vi "TCP IP Command Tester.vi"() -> ()   [LabVIEW 2024]
uses:
  Controls/Control_Fornax Set Monopolar Command - Coag Mode Enum.ctl
  Controls/Control_Fornax Set Monopolar Command - Serial Number String.ctl
  Controls/Control_Fornax Set Monopolar Command - Energy Channel ID Enum.ctl
  Controls/Control_Fornax Set Monopolar Command - Cut Mode Enum.ctl
  Controls/Control_Fornax Set Monopolar Command - Cut Power Command Enum.ctl
  Controls/Control_Fornax Set Monopolar Command - Coag Power Command Enum.ctl
  Program Files/National Instruments/LabVIEW 2024/examples/Design Patterns/Queued Message Handler/support/QMH Fundamentals - Message Cluster.ctl
panel:
  in  "Tab Control":enum32{"Page 1", "Page 2"}(tab)
  in  "error in (no error)":errorcluster
  out "output cluster":T1
  out "Array":T2(array[cluster])
  in  "Fornax Executable Path":path=path "C:/Program Files (x86)/Medtronic/Fornax/x86/Fornax.exe"
  in  "Action 1":bool
  in  "ExternalCommCommand":T3(ring)=enum."EXTERNAL_COMM_COMMAND_PAIR_INTEGRATION_TESTOR"
  in  "Stop":bool
  out "Display Message":string="Wait while TCP Connection established"
  in  "Set Monopolar Command":bool
  in  "CoagMode":T4
  in  "Serial Number":T5="T5G00443DX"
  in  "EnergyChannelID":T6
  in  "CutMode":T7
  in  "CutPowerCommand":T8
  in  "CoagPowerCommand":T9
  out "String":string
  in  "Numeric (0-8)":i32
  in  "Send String Command":bool
  out "status":bool
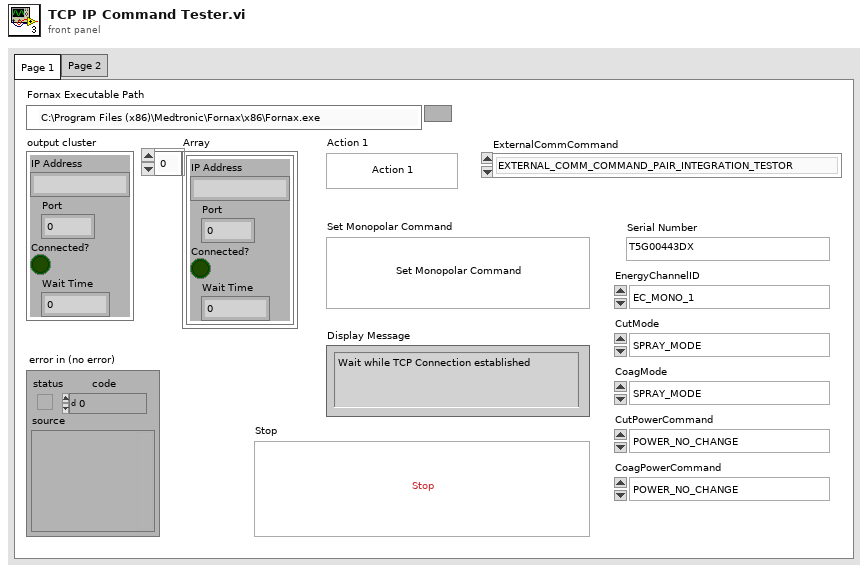
[diagram p1: front panel]
types:
  T1 = cluster{"IP Address":string, "Port":u16, "Connected?":bool, "Wait Time":dbl}
  T2 = cluster{"IP Address":string, "Port":u16, "Connected?":bool, "Wait Time":dbl}[]
  T3 = enum16{"EXTERNAL_COMM_COMMAND_INVALID", "EXTERNAL_COMM_COMMAND_PAIR_VLEX", "EXTERNAL_COMM_COMMAND_PAIR_FORNAX", "EXTERNAL_COMM_COMMAND_PAIR_INTEGRATION_TESTOR", "EXTERNAL_COMM_COMMAND_ENABLE_DFA", "EXTERNAL_COMM_COMMAND_ENABLE_DFT", "EXTERNAL_COMM_COMMAND_ENABLE_VIPER", "EXTERNAL_COMM_COMMAND_AUTO_ETHERNET_ON", "EXTERNAL_COMM_COMMAND_AUTO_ETHERNET_OFF", "EXTERNAL_COMM_COMMAND_STREAM_RFDATA_ON", "EXTERNAL_COMM_COMMAND_STREAM_RFDATA_OFF", "EXTERNAL_COMM_COMMAND_STREAM_ISOFIRM_ON", "EXTERNAL_COMM_COMMAND_STREAM_ISOFIRM_OFF", "EXTERNAL_COMM_COMMAND_STREAM_RFID_ON", "EXTERNAL_COMM_COMMAND_STREAM_RFID_OFF", "EXTERNAL_COMM_COMMAND_AUTO_ETHERNET_ONCE"}
  T4 = typedef "Control_Fornax Set Monopolar Command - Coag Mode Enum.ctl" = enum16{"SPRAY_MODE", "CUT_MODE", "BLEND_MODE", "FULGERATE_MODE", "BEPOLAR_MODE", "VESSEL_SEALING_MODE", "VALLEYLAB_MODE", "BIPOLAR_RESECTION_CUT_MODE", "BIPOLAR_RESECTION_COAG_MODE", "AUTOBIPOLAR_MODE", "VIPER_HLA", "SOFT_COAG_MODE", "NUM_ENERGY_MODES"}
  T5 = typedef "Control_Fornax Set Monopolar Command - Serial Number String.ctl" = string
  T6 = typedef "Control_Fornax Set Monopolar Command - Energy Channel ID Enum.ctl" = enum16{"EC_MONO_1", "EC_BIPOLAR", "EC_MONO_2", "EC_ADVANCED", "NUM_ENERGY_CHANNELS", "EC_NOT_USED"}
  T7 = typedef "Control_Fornax Set Monopolar Command - Cut Mode Enum.ctl" = enum16{"SPRAY_MODE", "CUT_MODE", "BLEND_MODE", "FULGERATE_MODE", "BIPOLAR_MODE", "VESSEL_SEALING_MODE", "VALLEYLAB_MODE", "BIPOLAR_RESECTION_CUT_MODE", "BIPOLAR_RESECTION_COAG_MODE", "AUTOBIPOLAR_MODE", "VIPER_HLA", "SOFT_COAG_MODE", "NUM_ENERGY_MODES"}
  T8 = typedef "Control_Fornax Set Monopolar Command - Cut Power Command Enum.ctl" = enum16{"POWER_NO_CHANGE", "POWER_INCREASE", "POWER_DECREASE", "POWER_INCREASE_REPEAT", "POWER_DECREASE_REPEAT"}
  T9 = typedef "Control_Fornax Set Monopolar Command - Coag Power Command Enum.ctl" = enum16{"POWER_NO_CHANGE", "POWER_INCREASE", "POWER_DECREASE", "POWER_INCREASE_REPEAT", "POWER_DECREASE_REPEAT"}
  T10 = typedef "QMH Fundamentals - Message Cluster.ctl" = cluster{"Message":string, "Message Data":variant}
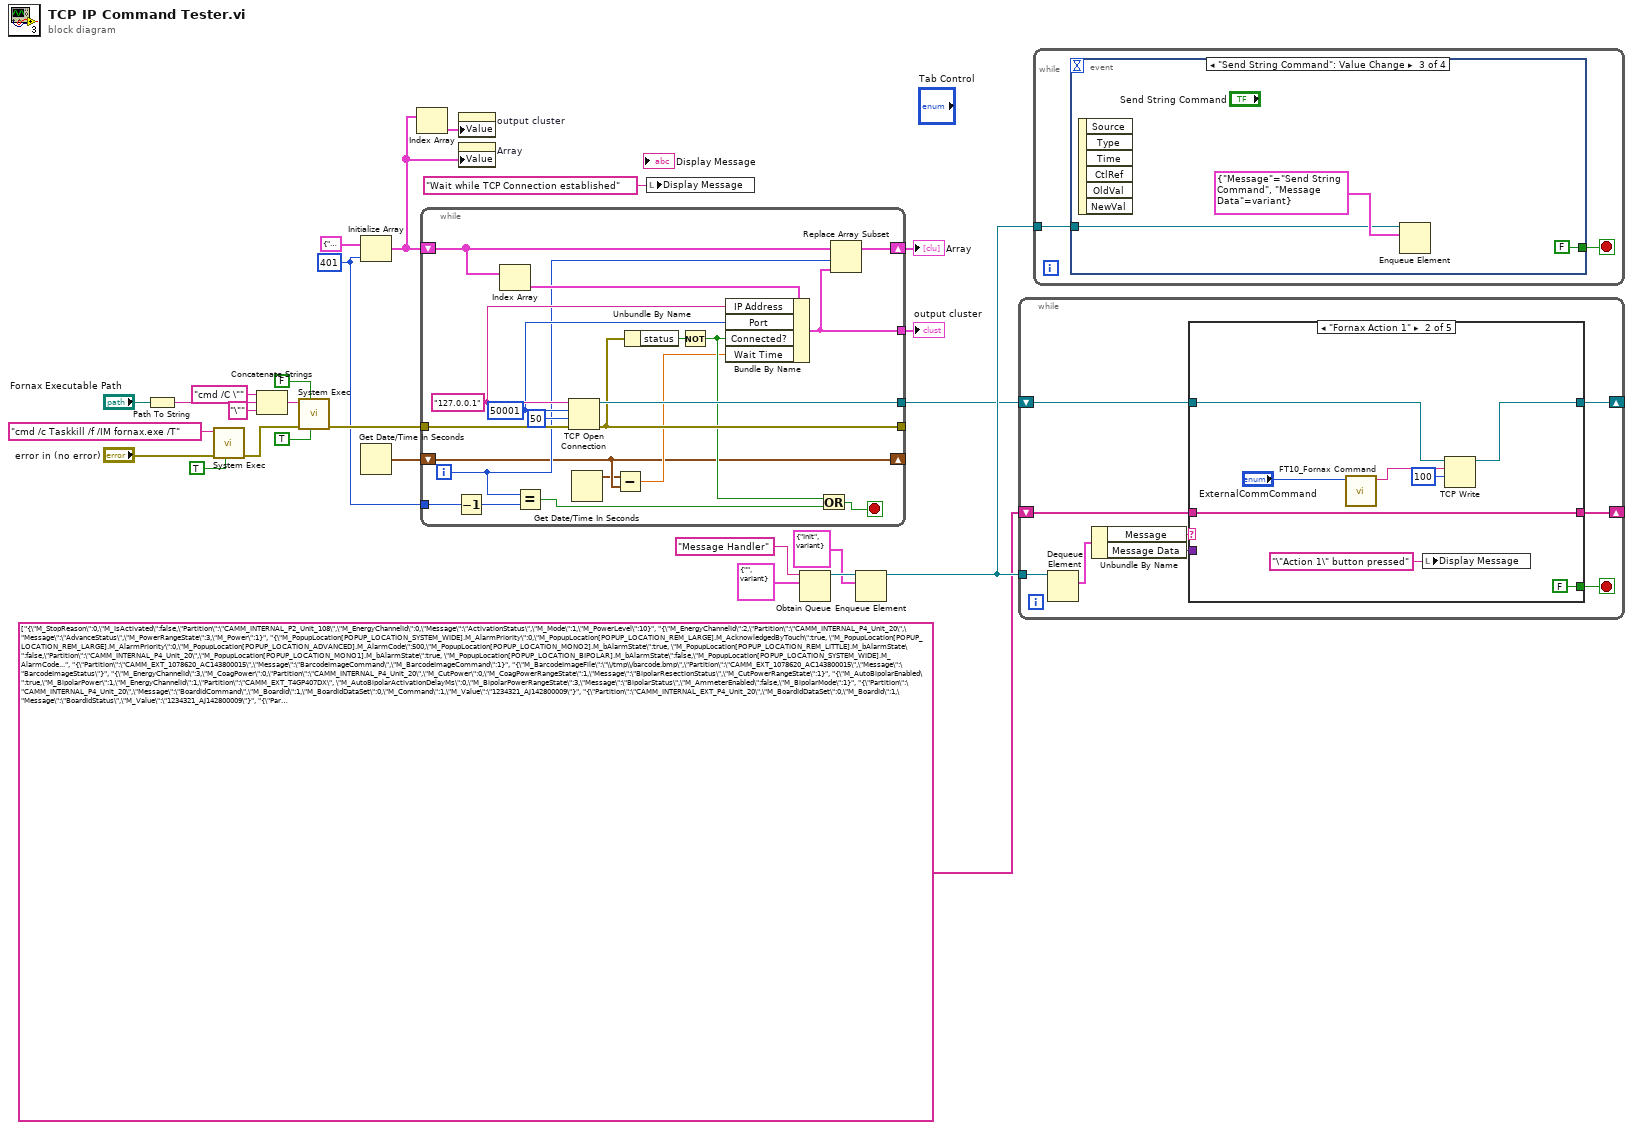
[diagram p0: block diagram]
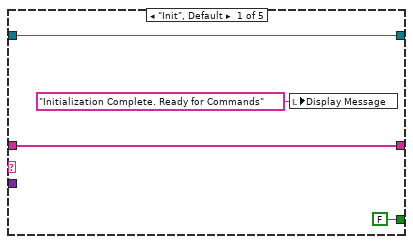
[diagram p2: hidden frame]
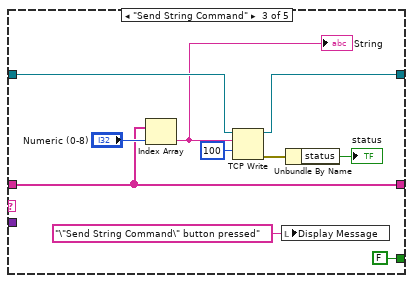
[diagram p3: hidden frame]
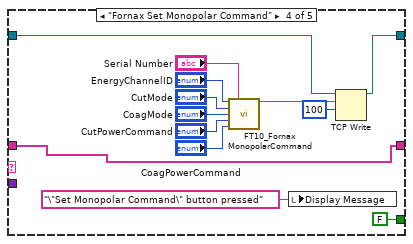
[diagram p4: hidden frame]
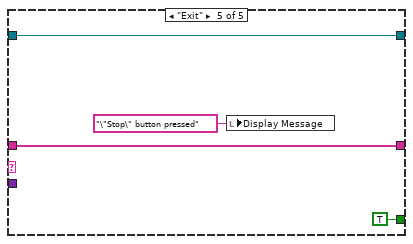
[diagram p5: hidden frame]
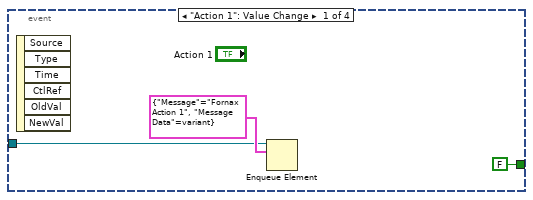
[diagram p6: hidden frame]
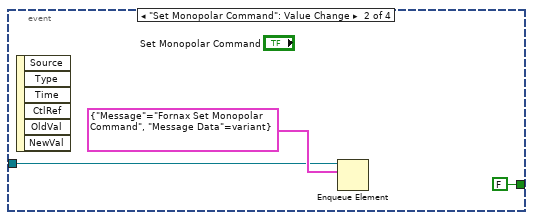
[diagram p7: hidden frame]
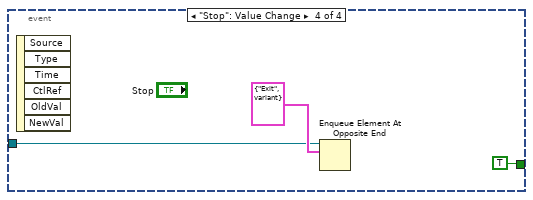
[diagram p8: hidden frame]
diagram:
  w24 = 401 ("dimension size")
  n1 = Path To String(path="Fornax Executable Path") -> (string=w13:string)
  n2 = call <vilib>:"System Exec.vi"("run minimized? (F)"=TRUE, "error in (no error)"="error in (no error)", "command line"="cmd /c Taskkill /f /IM fornax.exe /T") -> ("error out"=w19:errorcluster)  [unwired: 5 in, 3 out]
  n3 = Concatenate Strings("cmd /C \"" ("string"), w13, "\"" ("string")) -> (w15:string)
  n4 = call <vilib>:"System Exec.vi"("run minimized? (F)"=TRUE, "wait until completion? (T)"=FALSE, "error in (no error)"=w19, "command line"=w15) -> ("error out"=w27:errorcluster)  [unwired: 4 in, 3 out]
  n5 = Initialize Array(T1 {"IP Address"="", "Port"=0, "Connected?"=FALSE, "Wait Time"=0.0} ("Cluster"), w24) -> (w2:T2)
  n6 = Get Date/Time In Seconds() -> (seconds since 1Jan1904=w21:timestamp)
  n7 = Index Array(array=w2) -> (element=w3:T1)  [unwired: 1 in]
  n8 = while {
    tunnel: [w46] -> w5
    shift-right: [w45] -> w22
    shift-left: w2 -> [w44]
    tunnel: w24 -> [w35]
    tunnel: [w32] -> w23
    shift-right: [w29] -> _
    shift-left: w21 -> [w29]
    tunnel: w27 -> [w47]
    tunnel: [w40] -> _
    i -> [w31]
    stop <- w37 stop-if-true
    w41 = u16 50001 ("remote port or service name")
    w42 = "127.0.0.1" ("address")
    n9 = Decrement(x=w35) -> (x-1=w34:i32)
    n10 = Index Array(array=w44) -> (element=w43:T1)  [unwired: 1 in]
    n11 = Equal?(x=w31, y=w34) -> (x = y?=w33:bool)
    n12 = TCP Open Connection(address=w42, remote port or service name=w41, timeout ms (60000)=50, error in (no error)=w47) -> (connection ID=w46:refnum<k5>, error out=w40:errorcluster)  [unwired: 1 in]
    n13 = Get Date/Time In Seconds() -> (seconds since 1Jan1904=w28:timestamp)
    n14 = Subtract(x=w28, y=w29) -> (x-y=w30:dbl)
    n15 = Unbundle By Name(w40) -> ("status"=w39:bool)
    n16 = Not(x=w39) -> (.not. x?=w36:bool)
    n17 = Bundle By Name(cluster=w43, "IP Address"=w42, "Port"=w41, "Connected?"=w36, "Wait Time"=w30) -> (w32:T1)
    n18 = Or(x=w36, y=w33) -> (x .or. y?=w37:bool)
    n19 = Replace Array Subset(array=w44, new element=w32, index=w31) -> (w45:T2)
  }
  "output cluster" <- w23
  "Array" <- w22
  n20 = property on="output cluster" class="Clust (strict)"("Value"=w3) -> ()  [unwired: 2 in, 2 out]
  n21 = property on="Array" class="Arr (strict)"("Value"=w2) -> ()  [unwired: 2 in, 2 out]
  n22 = local write "Display Message"("Wait while TCP Connection established" ("Display Message")) -> ()
  n23 = Obtain Queue(name (unnamed)="Message Handler", element data type=T10 {"Message"="", "Message Data"=variant} ("Message Cluster")) -> (queue out=w9:refnum<queue>)  [unwired: 3 in, 2 out]
  n24 = Enqueue Element(queue=w9, element=T10 {"Message"="Init", "Message Data"=variant}) -> (queue out=w6:refnum<queue>)  [unwired: 2 in, 2 out]
  n25 = while {
    tunnel: w6 -> [w55]
    shift-right: [w52] -> _
    shift-left: w5 -> [w51]
    shift-right: [w49] -> _
    shift-left: string[] ["{\"M_StopReason\":0,\"M_IsActivated\":false,\"Partition\":\"CAMM_INTERNAL_P2_Unit_108\",\"M_EnergyChannelId\":0,\"Message\":\"ActivationStatus\",\"M_Mode\":1,\"M_PowerLevel\":10}", "{\"M_EnergyChannelId\":2,\"Partition\":\"CAMM_INTERNAL_P4_Unit_20\",\"Message\":\"AdvanceStatus\",\"M_PowerRangeState\":3,\"M_Power\":1}", "{\"M_PopupLocation[POPUP_LOCATION_SYSTEM_WIDE].M_AlarmPriority\":0,\"M_PopupLocation[POPUP_LOCATION_REM_LARGE].M_AcknowledgedByTouch\":true, \"M_PopupLocation[POPUP_LOCATION_REM_LARGE].M_AlarmPriority\":0,\"M_PopupLocation[POPUP_LOCATION_ADVANCED].M_AlarmCode\":500,\"M_PopupLocation[POPUP_LOCATION_MONO2].M_bAlarmState\":true, \"M_PopupLocation[POPUP_LOCATION_REM_LITTLE].M_bAlarmState\":false,\"Partition\":\"CAMM_INTERNAL_P4_Unit_20\",\"M_PopupLocation[POPUP_LOCATION_MONO1].M_bAlarmState\":true, \"M_PopupLocation[POPUP_LOCATION_BIPOLAR].M_bAlarmState\":false,\"M_PopupLocation[POPUP_LOCATION_SYSTEM_WIDE].M_AlarmCode\":500,\"M_PopupLocation[POPUP_LOCATION_DEMO_MODE].M_AlarmCode\":500, \"M_PopupLocation[POPUP_LOCATION_SYSTEM_WIDE].M_AcknowledgedByTouch\":true,\"M_PopupLocation[POPUP_LOCATION_ADVANCED].M_AcknowledgedByTouch\":true, \"M_PopupLocation[POPUP_LOCATION_REM_LARGE].M_bAlarmState\":false,\"M_PopupLocation[POPUP_LOCATION_REM_LITTLE].M_AcknowledgedByTouch\":false,\"M_PopupLocation[POPUP_LOCATION_BIPOLAR].M_AlarmCode\":500, \"M_PopupLocation[POPUP_LOCATION_MONO1].M_AcknowledgedByTouch\":true,\"M_PopupLocation[POPUP_LOCATION_MONO1].M_AlarmCode\":331,\"M_PopupLocation[POPUP_LOCATION_REM_LITTLE].M_AlarmPriority\":0, \"Message\":\"AlarmPopupStatus\",\"M_PopupLocation[POPUP_LOCATION_DEMO_MODE].M_AcknowledgedByTouch\":true,\"M_PopupLocation[POPUP_LOCATION_MONO2].M_AlarmCode\":331, \"M_PopupLocation[POPUP_LOCATION_ADVANCED].M_AlarmPriority\":0,\"M_PopupLocation[POPUP_LOCATION_REM_LITTLE].M_AlarmCode\":500,\"M_PopupLocation[POPUP_LOCATION_BIPOLAR].M_AcknowledgedByTouch\":true, \"M_PopupLocation[POPUP_LOCATION_MONO1].M_AlarmPriority\":3,\"M_PopupLocation[POPUP_LOCATION_REM_LARGE].M_AlarmCode\":500,\"M_PopupLocation[POPUP_LOCATION_DEMO_MODE].M_bAlarmState\":false, \"M_PopupLocation[POPUP_LOCATION_SYSTEM_WIDE].M_bAlarmState\":false,\"M_PopupLocation[POPUP_LOCATION_MONO2].M_AcknowledgedByTouch\":true, \"M_PopupLocation[POPUP_LOCATION_BIPOLAR].M_AlarmPriority\":0,\"M_PopupLocation[POPUP_LOCATION_ADVANCED].M_bAlarmState\":false, \"M_PopupLocation[POPUP_LOCATION_DEMO_MODE].M_AlarmPriority\":0,\"M_PopupLocation[POPUP_LOCATION_MONO2].M_AlarmPriority\":3}", "{\"Partition\":\"CAMM_EXT_1078620_AC143800015\",\"Message\":\"BarcodeImageCommand\",\"M_BarcodeImageCommand\":1}", "{\"M_BarcodeImageFile\":\"\\/tmp\\/barcode.bmp\",\"Partition\":\"CAMM_EXT_1078620_AC143800015\",\"Message\":\"BarcodeImageStatus\"}", "{\"M_EnergyChannelId\":3,\"M_CoagPower\":0,\"Partition\":\"CAMM_INTERNAL_P4_Unit_20\",\"M_CutPower\":0,\"M_CoagPowerRangeState\":1,\"Message\":\"BipolarResectionStatus\",\"M_CutPowerRangeState\":1}", "{\"M_AutoBipolarEnabled\":true,\"M_BipolarPower\":1,\"M_EnergyChannelId\":1,\"Partition\":\"CAMM_EXT_T4GP407DX\", \"M_AutoBipolarActivationDelayMs\":0,\"M_BipolarPowerRangeState\":3,\"Message\":\"BipolarStatus\",\"M_AmmeterEnabled\":false,\"M_BipolarMode\":1}", "{\"Partition\":\"CAMM_INTERNAL_P4_Unit_20\",\"Message\":\"BoardIdCommand\",\"M_BoardId\":1,\"M_BoardIdDataSet\":0,\"M_Command\":1,\"M_Value\":\"1234321_AJ142800009\"}", "{\"Partition\":\"CAMM_INTERNAL_EXT_P4_Unit_20\",\"M_BoardIdDataSet\":0,\"M_BoardId\":1,\"Message\":\"BoardIdStatus\",\"M_Value\":\"1234321_AJ142800009\"}", "{\"Partition\":\"CAMM_INTERNAL_EXT_P4_Unit_20\",\"Message\":\"CardioblateBipolarStatus\",\"M_EnergyChannelId\":3,\"M_MaximumAblationTimeMS\":5,\"M_MaximumPowerLevel\":5}", "{\"Partition\":\"CAMM_INTERNAL_EXT_P4_Unit_20\",\"Message\":\"CardioblateMonopolarStatus\",\"M_CardioblateMonopolarPower\":5, \"M_CardioblateMonopolarPowerRangeState\":3,\"M_MaximumActivationTimeMS\":10,\"M_MaximumActivationTimeMSRangeState\":3}", "{\"Partition\":\"CAMM_INTERNAL_EXT_P4_Unit_20\",\"Message\":\"CardioblateSelectStatus\",\"M_SelectedEnergyChannel\":3}", "{\"Partition\":\"CAMM_EXT_1078620_AC143800015\",\"Message\":\"DftAlarmCommand\",\"M_ModuleId\":21,\"M_AlarmCode\":331, \"M_Command\":4,\"M_EnergyChannelId\":0,\"M_Message\":\"HELP\", \"M_CommandParams\":\"\",\"M_CommandOptions\":\"\"}", "{\"Partition\":\"CAMM_INTERNAL_EXT_P4_Unit_20\",\"M_AudioSequence\":1,\"Message\":\"DftAudioPlayCommand\",\"M_PlayMode\":3,\"M_Priority\":0,\"M_Volume\":50,\"M_OverrideSeqVolume\":false}", "{\"M_EnergyChannelId\":3,\"Partition\":\"CAMM_INTERNAL_EXT_P4_Unit_20\",\"Message\":\"DftInstrumentCommand\",\"M_DftInstrumentCommand\":1,\"M_IntValue\":0,\"M_FloatValue\":0.0,\"M_StringValue\":\"\"}", "{\"Partition\":\"CAMM_EXT_1078620_AC143800015\",\"Message\":\"DftLogCommand\",\"M_Command\":3,\"M_CommandOptions\":\"\"}", "{\"M_Command\":1,\"M_CalibrationType\":0,\"M_CalibrationTime\":\"\",\"M_Options\":\"\",\"M_EmA2dCalData.M_BipLowCurrentSecondary.M_Offset\":0.0,\"M_EmA2dCalData.M_BipLowCurrentPrimary.M_Gain\":1.0, \"M_EmA2dCalData.M_BipLowVoltPrimary.M_Gain\":1.0,\"Partition\":\"CAMM_INTERNAL_EXT_P4_Unit_20\",\"M_EmA2dCalData.M_BipHighVoltSecondary.M_Offset\":0.0,\"M_EmA2dCalData.M_BipLowVoltSecondary.M_Gain\":1.0, \"M_EmA2dCalData.M_BipLowVoltPrimary.M_Offset\":0.0,\"M_EmA2dCalData.M_BipHighVoltPrimary.M_Gain\":1.0,\"M_EmA2dCalData.M_MonoLowVoltPrimary.M_Offset\":0.0, \"M_EmA2dCalData.M_MonoLowVoltSecondary.M_Offset\":0.0,\"M_EmA2dCalData.M_BipHighCurrentSecondary.M_Offset\":0.0,\"M_EmA2dCalData.M_MonoLowVoltSecondary.M_Gain\":1.0, \"M_EmA2dCalData.M_BipHighCurrentPrimary.M_Gain\":1.0,\"M_EmA2dCalData.M_BipHighVoltSecondary.M_Gain\":1.0,\"M_EmA2dCalData.M_MonoHighVoltSecondary.M_Offset\":0.0, \"M_EmA2dCalData.M_BipHighCurrentPrimary.M_Offset\":0.0,\"Message\":\"EmA2dCalDataCommand\",\"M_EmA2dCalData.M_BipLowCurrentSecondary.M_Gain\":1.0, \"M_EmA2dCalData.M_BipLowCurrentPrimary.M_Offset\":0.0,\"M_EmA2dCalData.M_MonoHighVoltPrimary.M_Gain\":1.0, \"M_EmA2dCalData.M_BipHighCurrentSecondary.M_Gain\":1.0,\"M_EmA2dCalData.M_MonoHighVoltSecondary.M_Gain\":1.0, \"M_EmA2dCalData.M_BipHighVoltPrimary.M_Offset\":0.0,\"M_EmA2dCalData.M_MonoLowVoltPrimary.M_Gain\":1.0, \"M_EmA2dCalData.M_MonoHighVoltPrimary.M_Offset\":0.0,\"M_EmA2dCalData.M_BipLowVoltSecondary.M_Offset\":0.0}", "{\"M_EmA2dCalData.M_BipLowCurrentSecondary.M_Offset\":0.0,\"M_EmA2dCalData.M_BipLowCurrentPrimary.M_Gain\":1.01491,\"M_EmA2dCalData.M_BipLowVoltPrimary.M_Gain\":1.03926, \"Partition\":\"CAMM_EXT_1078620_AC143800029\",\"M_EmA2dCalData.M_BipHighVoltSecondary.M_Offset\":0.0,\"M_EmA2dCalData.M_BipLowVoltPrimary.M_Offset\":0.0, \"M_EmA2dCalData.M_BipLowVoltSecondary.M_Gain\":1.02606,\"M_EmA2dCalData.M_BipHighVoltPrimary.M_Gain\":1.03662,\"M_EmA2dCalData.M_MonoLowVoltPrimary.M_Offset\":0.0, \"M_EmA2dCalData.M_MonoLowVoltSecondary.M_Offset\":0.0,\"M_EmA2dCalData.M_BipHighCurrentSecondary.M_Offset\":0.0,\"M_EmA2dCalData.M_MonoLowVoltSecondary.M_Gain\":1.05138, \"M_EmA2dCalData.M_BipHighCurrentPrimary.M_Gain\":1.01475,\"M_EmA2dCalData.M_BipHighVoltSecondary.M_Gain\":1.02351,\"M_EmA2dCalData.M_MonoHighVoltSecondary.M_Offset\":0.0, \"M_EmA2dCalData.M_BipHighCurrentPrimary.M_Offset\":0.0,\"Message\":\"EmA2dCalDataStatus\",\"M_EmA2dCalData.M_BipLowCurrentSecondary.M_Gain\":1.0347, \"M_EmA2dCalData.M_BipLowCurrentPrimary.M_Offset\":0.0,\"M_EmA2dCalData.M_MonoHighVoltPrimary.M_Gain\":1.07264,\"M_EmA2dCalData.M_MonoHighVoltSecondary.M_Gain\":1.05568, \"M_EmA2dCalData.M_BipHighCurrentSecondary.M_Gain\":1.03478,\"M_Options\":\"\",\"M_EmA2dCalData.M_BipHighVoltPrimary.M_Offset\":0.0, \"M_CalibrationTime\":\"2014-11-18T00:26:27Z\", \"M_EmA2dCalData.M_MonoLowVoltPrimary.M_Gain\":1.06396,\"M_EmA2dCalData.M_MonoHighVoltPrimary.M_Offset\":0.0, \"M_CalibrationType\":-1,\"M_EmA2dCalData.M_BipLowVoltSecondary.M_Offset\":0.0}", "{\"Message\":\"EnergyParameterCommand\",\"Partition\":\"CAMM_EXT_1078620_AC143800015\",\"M_EnergyChannelId\":0;,\"M_InstrumentType\":1;,\"M_ParameterType\":1,\"M_ParameterValue\":3,\"M_EnergyMode\":-1}", "{\"Message\":\"ExternalCommCommand\",\"Partition\":\"CAMM_EXT_1078620_AC143800015\",\"M_ControllerBoardId\":\"1078620_AC143800015\",\"M_ClientId\":\"\",\"M_Command\":5,\"M_CommandOptions\":\"\"}"] ("String") -> [w48]
    stop <- w50 stop-if-true
    n26 = Dequeue Element(queue=w55) -> (element=w56:T10)  [unwired: 2 in, 3 out]
    n27 = Unbundle By Name(w56) -> ("Message"=w54:string, "Message Data"=w53:variant)
    n28 = case shown="\"Fornax Action 1\"" w54 {
      tunnel: w53 -> [_ _ _ _ _]
      tunnel: [w60 w64 w77 w89 w93] -> w52
      tunnel: w51 -> [w60 w65 w78 w90 w93]
      tunnel: [FALSE FALSE FALSE FALSE TRUE] -> w50
      tunnel: [w57 w61 w73 w79 w92] -> w49
      tunnel: w48 -> [w57 w61 w73 w79 w92]
      frame "Init", Default {
        n29 = local write "Display Message"("Initialization Complete. Ready for Commands" ("Display Message")) -> ()
      }
      frame "Fornax Action 1" {
        n30 = call "FT10_Fornax Command.vi"("ExternalCommCommand"="ExternalCommCommand") -> ("JSON Message"=w67:string)  [unwired: 10 in]
        n31 = local write "Display Message"("\"Action 1\" button pressed" ("Display Message")) -> ()
        n32 = TCP Write(connection ID=w65, data in=w67, 9:100 ("timeout ms (25000)")) -> (connection ID out=w64:refnum<k5>)  [unwired: 1 in, 2 out]
      }
      frame "Send String Command" {
        n33 = Index Array(array=w73, index="Numeric (0-8)") -> (element=w69:string)
        "String" <- w69
        n34 = TCP Write(connection ID=w78, data in=w69, 9:100 ("timeout ms (25000)")) -> (connection ID out=w77:refnum<k5>, error out=w71:errorcluster)  [unwired: 1 in, 1 out]
        n35 = local write "Display Message"("\"Send String Command\" button pressed" ("Display Message")) -> ()
        n36 = Unbundle By Name(w71) -> ("status"=→"status":bool)
      }
      frame "Fornax Set Monopolar Command" {
        n37 = call "FT10_Fornax MonopolarCommand.vi"("EnergyChannelID"="EnergyChannelID", "Serial Number"="Serial Number", "CutMode"="CutMode", "CoagMode"="CoagMode", "CutPowerCommand"="CutPowerCommand", "CoagPowerCommand"="CoagPowerCommand") -> ("JSON Command"=w86:string)  [unwired: 9 in]
        n38 = local write "Display Message"("\"Set Monopolar Command\" button pressed" ("Display Message")) -> ()
        n39 = TCP Write(connection ID=w90, data in=w86, 9:100 ("timeout ms (25000)")) -> (connection ID out=w89:refnum<k5>)  [unwired: 1 in, 2 out]
      }
      frame "Exit" {
        n40 = local write "Display Message"("\"Stop\" button pressed" ("Display Message")) -> ()
      }
    }
  }
  n41 = while {
    tunnel: w6 -> [w97]
    stop <- w96 stop-if-true
    n42 = event shown="[2] \"Send String Command\": Value Change" {
      selector: _ -> [_ _ _ _]
      dyn-events: _ -> [_ _ _ _]
      timeout: _ -> [_ _ _ _]
      tunnel: w97 -> [w99 w102 w105 w108]
      tunnel: [FALSE FALSE FALSE TRUE] -> w96
      event "Action 1": Value Change {
        n43 = event-data() -> ()  [unwired: 1 in, 6 out]
        n44 = Enqueue Element(queue=w99, element=T10 {"Message"="Fornax Action 1", "Message Data"=variant}) -> ()  [unwired: 2 in, 3 out]
      }
      event "Set Monopolar Command": Value Change {
        n45 = event-data() -> ()  [unwired: 1 in, 6 out]
        n46 = Enqueue Element(queue=w102, element=T10 {"Message"="Fornax Set Monopolar Command", "Message Data"=variant}) -> ()  [unwired: 2 in, 3 out]
      }
      event "Send String Command": Value Change {
        n47 = event-data() -> ()  [unwired: 1 in, 6 out]
        n48 = Enqueue Element(queue=w105, element=T10 {"Message"="Send String Command", "Message Data"=variant}) -> ()  [unwired: 2 in, 3 out]
      }
      event "Stop": Value Change {
        n49 = event-data() -> ()  [unwired: 1 in, 6 out]
        n50 = Enqueue Element At Opposite End(queue=w108, element=T10 {"Message"="Exit", "Message Data"=variant}) -> ()  [unwired: 2 in, 3 out]
      }
    }
  }
